vi "c_Set Receiving Case.vi"() -> (1 "Case Label":T1)   [LabVIEW 2023, in "Message Pump.lvclass"]
uses:
  Message Pump.lvclass
  <vilib>/addons/_Workers/Library/Case Label.ctl
  <vilib>/addons/_Workers/Library/Workers.lvlib
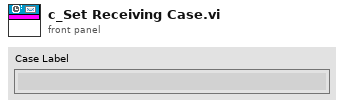
[diagram p1: front panel]
types:
  T1 = typedef "WORKERS.lvlib/Case Label.ctl" = string
  T2 = typedef "Workers.lvlib/Case Label.ctl" = string
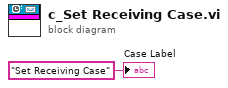
[diagram p0: block diagram]
diagram:
  "Case Label" <- T2 "Set Receiving Case" ("Case Label")
